vi "XNET Database Get DBC Attribute (ECU).vi"(0 "ECU in":refnum<k21>, 1 "mode":T1 items=["Attribute Value", "Enumeration", "Attribute Name List", "Signal Value Table"], 5 "attribute name":string, 11 "error in (no error)":errorcluster) -> (4 "ECU out":refnum<k21>, 8 "attribute text":string, 10 "is default?":bool=TRUE, 15 "error out":errorcluster)   [LabVIEW 2018]
doc: "Reads the specified attribute value from a DBC file.\nMode is an optional input that specifies the type of text to get."
uses:
  XNET Get DBC Mode.ctl
  nixlvapi.dll
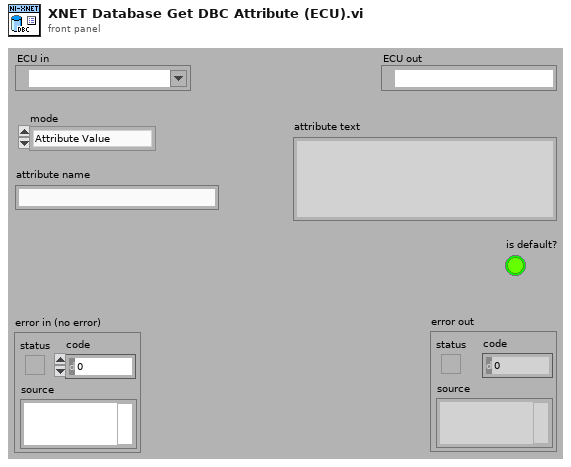
[diagram p1: front panel]
types:
  T1 = typedef "XNET Get DBC Mode.ctl" = u32
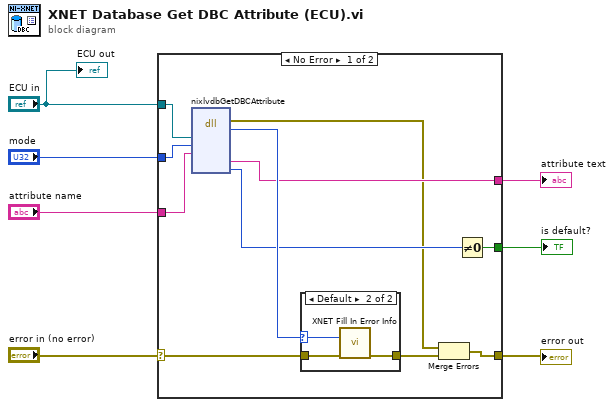
[diagram p0: block diagram]
diagram:
  n1 = case shown="No Error" "error in (no error)" {
    selector: "error in (no error)" -> [w17 w23]
    tunnel: [w9 w23] -> w7
    tunnel: "attribute name" -> [w15 _]
    tunnel: [w14 _] -> w4
    tunnel: [w13 _] -> w3
    tunnel: "ECU in" -> [w11 _]
    tunnel: "mode" -> [w10 _]
    frame No Error {
      n2 = dll-call lib="nixlvapi.*" fn="nixlvdbGetDBCAttribute" ("nilvxaiu.dll:lvxenDatabaseDeleteObject")("reference"=w11, "mode"=w10, "attributeName"=w15) -> (error out=w8:errorcluster, "return type"=w16:i32, "attributeText"=w14:string, "isDefault"=w12:u32)  [unwired: 5 in, 4 out]
      n3 = case shown="Default" w16 {
        selector: w16 -> [_ w20]
        tunnel: w17 -> [w19 w21]
        tunnel: [w19 w22] -> w18
        frame 0 {
        }
        frame Default {
          n4 = call "XNET Fill In Error Info.vi"("status code"=w20, "error in"=w21) -> ("error out"=w22:errorcluster)  [unwired: 13 out]
        }
      }
      n5 = Merge Errors(w8, w18) -> (w9:errorcluster)
      n6 = Not Equal To 0?(x=w12) -> (x != 0?=w13:bool)
    }
    frame Error {
    }
  }
  "error out" <- w7
  "attribute text" <- w4
  "is default?" <- w3
  "ECU out" <- "ECU in"
